vi "Part 2.vi"(11 "Input":string) -> (3 "Output":i64)   [LabVIEW 2021]
uses:
  dece495d-f556-4a12-9819-8aa362c7f80d.vi
  <userlib>/_OpenG.lib/string/string.llb/Convert EOLs (String)__ogtk.vi
  1846c71f-6748-4b9f-a217-25f6b413c366.vi
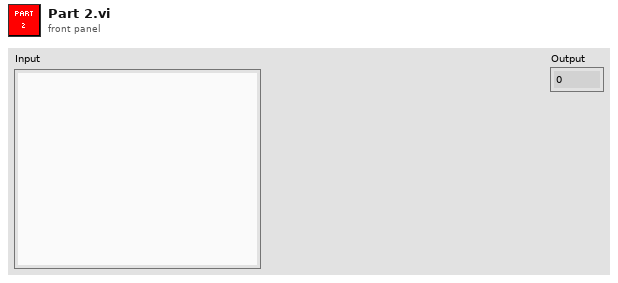
[diagram p1: front panel]
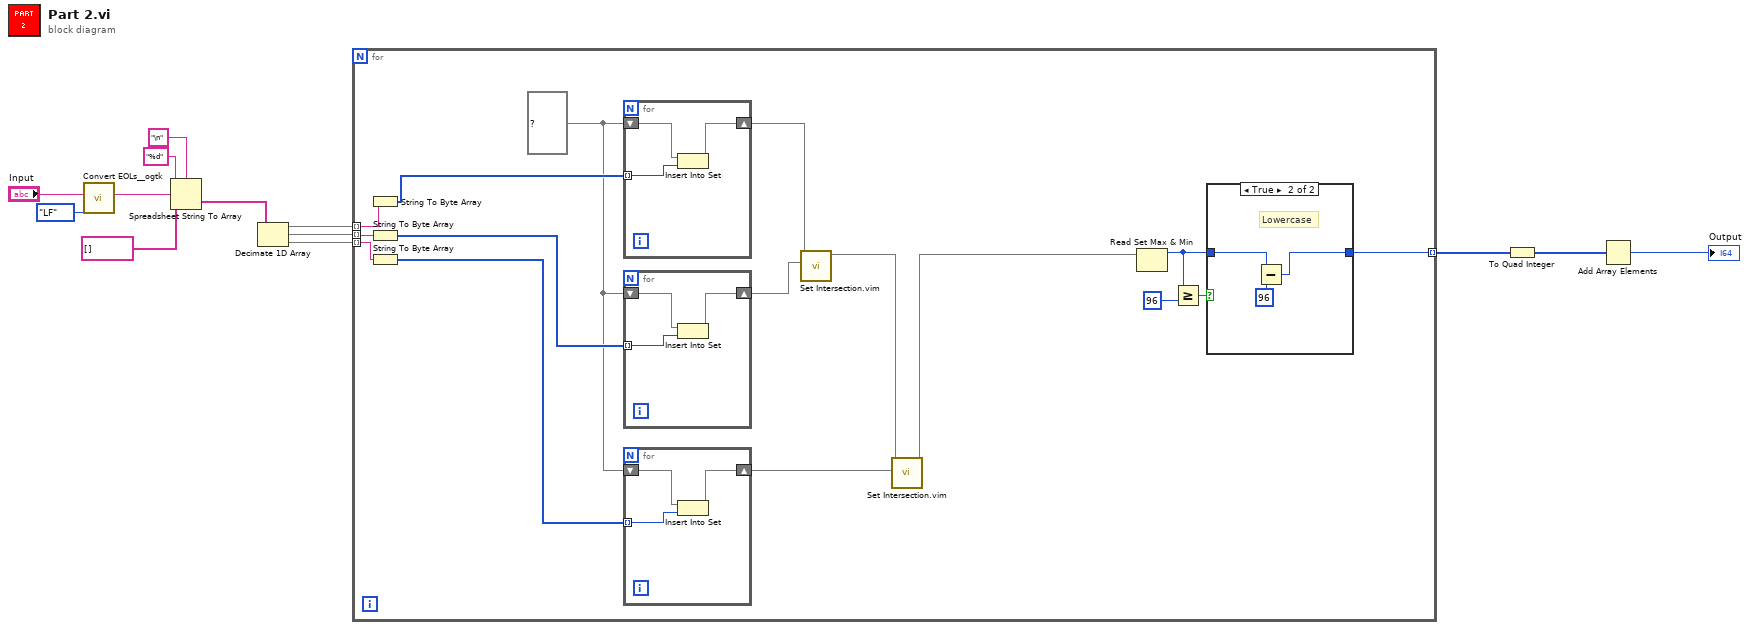
[diagram p0: block diagram]
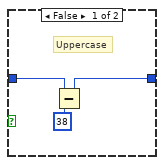
[diagram p2: hidden frame]
diagram:
  n1 = call-poly <userlib>:"Convert EOLs__ogtk.vi"("Convert to:"=enum16{"CR", "LF", "CRLF"}."LF", "String in"="Input") -> ("String out"=w6:string)  [unwired: 9 in]
  n2 = Spreadsheet String To Array(delimiter (Tab)="\n", format string="%d", spreadsheet string=w6, array type (2D Dbl)=string[] []) -> (array=w4:string[])
  n3 = Decimate 1D Array(w4) -> (w3:string[], w2:string[], w1:string[])
  n4 = for {
    tunnel: [w24] -> w9 mode=indexing
    tunnel: w3 -> [w22] mode=indexing
    tunnel: w2 -> [w21] mode=indexing
    tunnel: w1 -> [w20] mode=indexing
    w18 = set{u8} {} ("set in")
    n5 = String To Byte Array(string=w22) -> (unsigned byte array=w23:u8[])
    n6 = String To Byte Array(string=w21) -> (unsigned byte array=w19:u8[])
    n7 = String To Byte Array(string=w20) -> (unsigned byte array=w17:u8[])
    n8 = for {
      tunnel: w23 -> [w44] mode=indexing
      shift-right: [w42] -> w29
      shift-left: w18 -> [w43]
      n9 = Insert Into Set(10:w44, 11:w43) -> (3:w42:set{u8})  [unwired: 1 out]
    }
    n10 = for {
      tunnel: w19 -> [w41] mode=indexing
      shift-right: [w39] -> w28
      shift-left: w18 -> [w40]
      n11 = Insert Into Set(10:w41, 11:w40) -> (3:w39:set{u8})  [unwired: 1 out]
    }
    n12 = for {
      tunnel: w17 -> [w32] mode=indexing
      shift-right: [w30] -> w16
      shift-left: w18 -> [w31]
      n13 = Insert Into Set(10:w32, 11:w31) -> (3:w30:set{u8})  [unwired: 1 out]
    }
    n14 = call "Set Intersection.vim"("set 2"=w28, "set 1"=w29) -> ("intersection"=w15:set{u8})  [unwired: 9 in]
    n15 = call "Set Intersection.vim"("set 2"=w16, "set 1"=w15) -> ("intersection"=w14:set{u8})  [unwired: 9 in]
    n16 = Read Set Max & Min(11:w14) -> (3:w25:u8)  [unwired: 1 out]
    n17 = Greater Or Equal?(x=w25, y=u8 96) -> (x >= y?=w27:bool)
    n18 = case shown="True" w27 {
      tunnel: w25 -> [w34 w36]
      tunnel: [w33 w37] -> w24
      frame False {
        # "Uppercase"
        n19 = Subtract(x=w34, y=u8 38) -> (x-y=w33:u8)
      }
      frame True {
        # "Lowercase"
        n20 = Subtract(x=w36, y=u8 96) -> (x-y=w37:u8)
      }
    }
  }
  n21 = To Quad Integer(1:w9) -> (0:w7:i64[])
  n22 = Add Array Elements(numeric array=w7) -> (sum=→"Output":i64)
